vi "Linspace(sub).vi"(1 "N of Steps":i32, 2 "End":dbl, 3 "Start":dbl) -> (0 "Array":dbl[](array[numeric]))   [LabVIEW 2009]
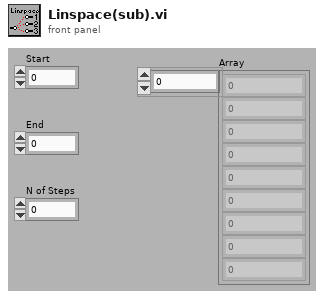
[diagram p1: front panel]
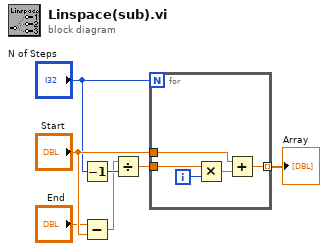
[diagram p0: block diagram]
diagram:
  n1 = Decrement(x="N of Steps") -> (x-1=w4:i32)
  n2 = Subtract(x="End", y="Start") -> (x-y=w2:dbl)
  n3 = Divide(x=w2, y=w4) -> (x/y=w1:dbl)
  n4 = for {
    N: "N of Steps" -> [_]
    tunnel: w1 -> [w10]
    tunnel: [w12] -> w6 mode=indexing
    tunnel: "Start" -> [w9]
    i -> [w11]
    n5 = Multiply(x=w10, y=w11) -> (x*y=w8:dbl)
    n6 = Add(x=w9, y=w8) -> (x+y=w12:dbl)
  }
  "Array" <- w6
